vi "IR2LambdaTemp.vi"(6 "SensorUsed":T1, 7 "VS feedback":dbl[](array[numeric]), 8 "error constant":errorcluster, 11 "VS control":dbl[](array[numeric])) -> (0 "error constant out":errorcluster, 3 "VS control out":dbl[](array[numeric]))   [LabVIEW 2017, in "ALMA_10201-10401_O2SensorSim Engine.lvlib"]
uses:
  ALMA_10201-10401_O2SensorSim Engine.lvlib
  Sensor_used.ctl
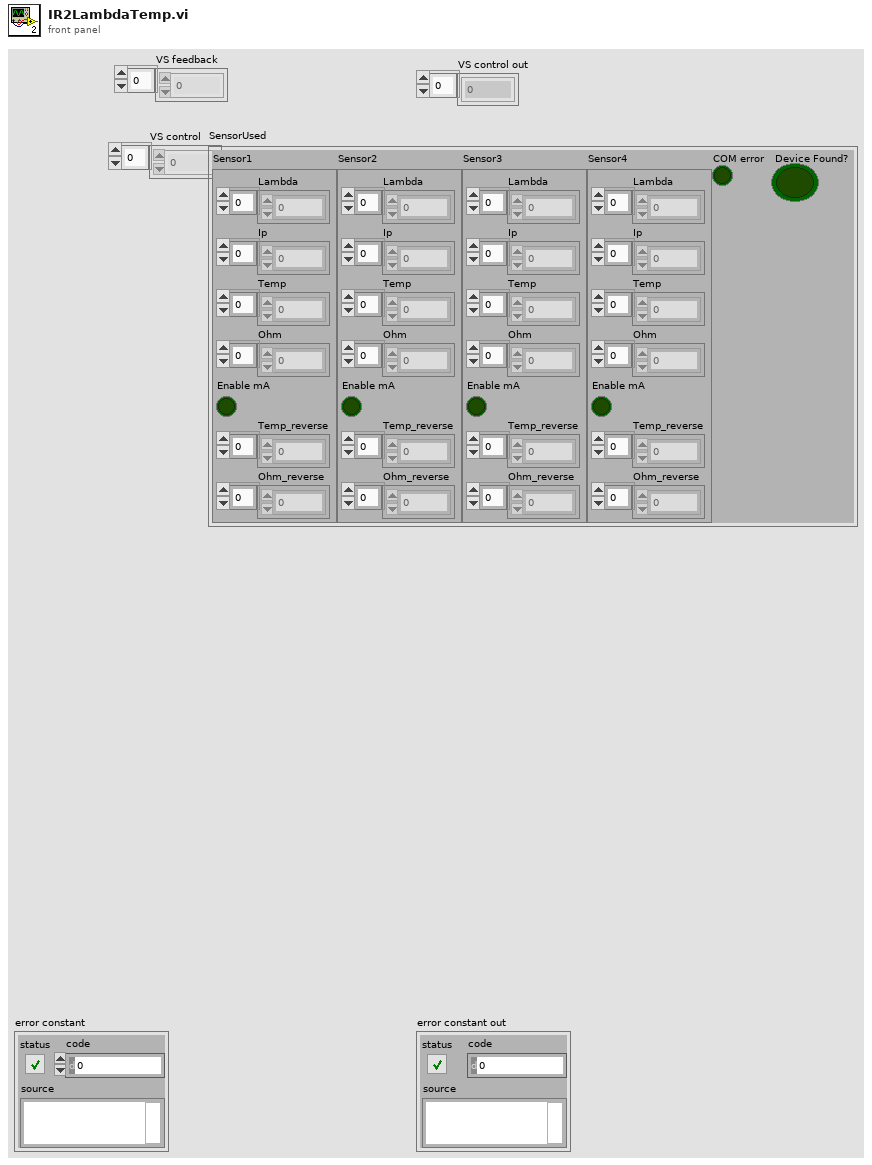
[diagram p1: front panel]
types:
  T1 = typedef "ALMA_10201-10401_O2SensorSim Engine.lvlib/Sensor_used.ctl" = cluster{"Sensor1":cluster{"Lambda":dbl[], "Ip":dbl[], "Temp":dbl[], "Ohm":dbl[], "Enable mA":bool, "Temp_reverse":dbl[], "Ohm_reverse":dbl[]}, "Sensor2":cluster{"Lambda":dbl[], "Ip":dbl[], "Temp":dbl[], "Ohm":dbl[], "Enable mA":bool, "Temp_reverse":dbl[], "Ohm_reverse":dbl[]}, "Sensor3":cluster{"Lambda":dbl[], "Ip":dbl[], "Temp":dbl[], "Ohm":dbl[], "Enable mA":bool, "Temp_reverse":dbl[], "Ohm_reverse":dbl[]}, "Sensor4":cluster{"Lambda":dbl[], "Ip":dbl[], "Temp":dbl[], "Ohm":dbl[], "Enable mA":bool, "Temp_reverse":dbl[], "Ohm_reverse":dbl[]}, "COM error":bool, "Device Found?":bool}
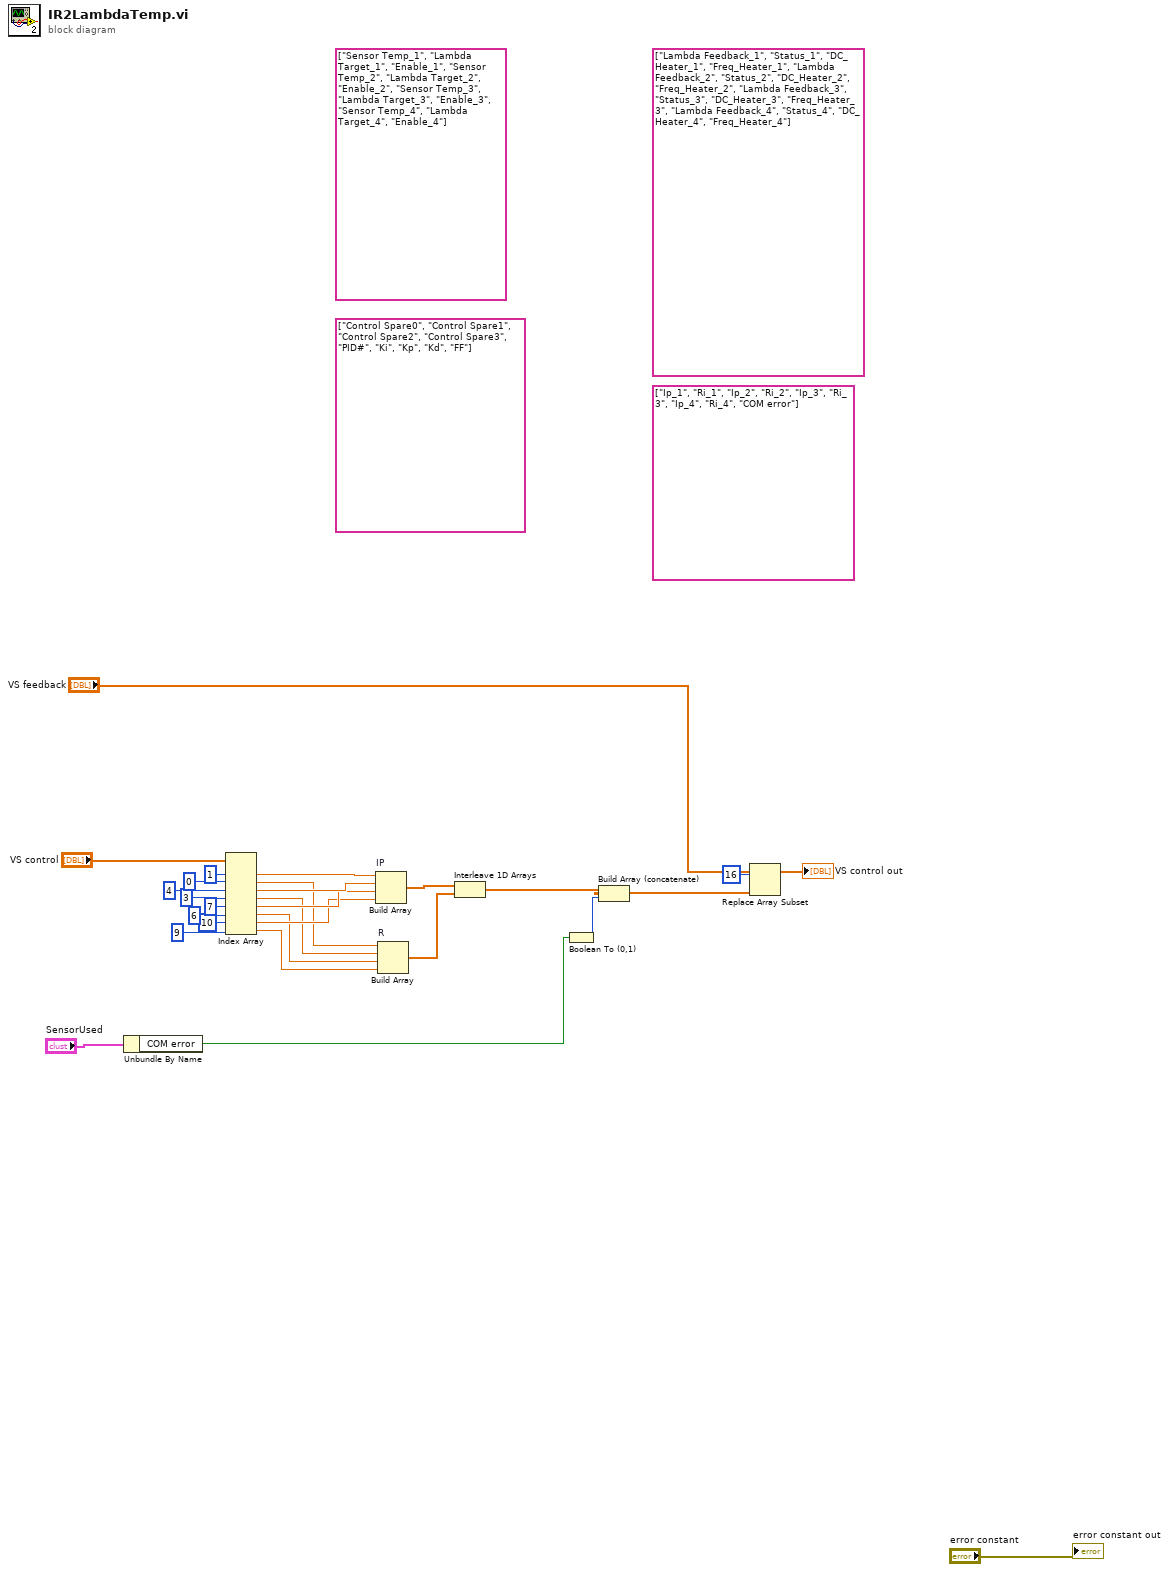
[diagram p0: block diagram]
diagram:
  (unwired) string[] ["Control Spare0", "Control Spare1", "Control Spare2", "Control Spare3", "PID#", "Ki", "Kp", "Kd", "FF"] ("Additional Control")
  (unwired) string[] ["Ip_1", "Ri_1", "Ip_2", "Ri_2", "Ip_3", "Ri_3", "Ip_4", "Ri_4", "COM error"] ("O2SensoSim Feedback 3")
  (unwired) string[] ["Lambda Feedback_1", "Status_1", "DC_Heater_1", "Freq_Heater_1", "Lambda Feedback_2", "Status_2", "DC_Heater_2", "Freq_Heater_2", "Lambda Feedback_3", "Status_3", "DC_Heater_3", "Freq_Heater_3", "Lambda Feedback_4", "Status_4", "DC_Heater_4", "Freq_Heater_4"] ("O2SensoSim Feedback 4")
  (unwired) string[] ["Sensor Temp_1", "Lambda Target_1", "Enable_1", "Sensor Temp_2", "Lambda Target_2", "Enable_2", "Sensor Temp_3", "Lambda Target_3", "Enable_3", "Sensor Temp_4", "Lambda Target_4", "Enable_4"] ("O2SensoSim Setpoint 2")
  n1 = Unbundle By Name("SensorUsed") -> ("COM error"=w1:bool)
  n2 = Index Array(array="VS control", index #1=1 ("index"), index #2=0 ("index"), index #3=4 ("index"), index #4=3 ("index"), index #5=7 ("index"), index #6=6 ("index"), index #7=10 ("index"), index #8=9 ("index")) -> (element #1=w10:dbl, element #2=w6:dbl, element #3=w9:dbl, element #4=w5:dbl, element #5=w8:dbl, element #6=w4:dbl, element #7=w7:dbl, element #8=w3:dbl)
  n3 = Build Array "IP"(w10, w9, w8, w7) -> (w18:dbl[])
  n4 = Build Array "R"(w6, w5, w4, w3) -> (w17:dbl[])
  n5 = Interleave 1D Arrays(w18, w17) -> (w14:dbl[])
  n6 = Boolean To (0,1)(Boolean=w1) -> (0, 1=w12:i16)
  n7 = Build Array (concatenate)(w14, w12) -> (w13:dbl[])
  n8 = Replace Array Subset(array="VS feedback", new element=w13, index=16) -> (→"VS control out":dbl[])
  "error constant out" <- "error constant"
